vi "Math-Is Bit Set.vi"(1 "Bit":i32=1, 2 "Integer":i32=3) -> (0 "Is Bit Set?":bool)   [LabVIEW 2020]
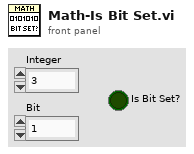
[diagram p1: front panel]
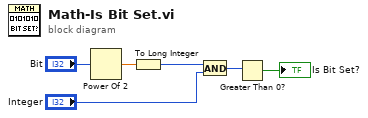
[diagram p0: block diagram]
diagram:
  n1 = Power Of 2(x="Bit") -> (2^x=w2:dbl)
  n2 = To Long Integer(number=w2) -> (32bit integer=w1:i32)
  n3 = And(x=w1, y="Integer") -> (x .and. y?=w6:i32)
  n4 = Greater Than 0?(x=w6) -> (x > 0?=→"Is Bit Set?":bool)
